vi "全局变量.vi"() -> ()   [LabVIEW 2018]
panel:
  in  "波特率":u32=115200
  in  "每次发送大小":i32=102400
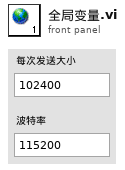
[diagram p1: front panel]
diagram:
